vi "F Dwf Analog Out Amplitude Info.vi"(7 "pvoltsMax":dbl, 8 "error in (no error)":errorcluster, 9 "pvoltsMin":dbl, 10 "idxChannel":i32, 11 "hdwf":i32) -> (0 "error out":errorcluster, 1 "pvoltsMin out":dbl, 3 "function return":i32, 5 "pvoltsMax out":dbl)   [LabVIEW 2019, in "Olasdwf.lvlib"]
doc: "DWFAPI int FDwfAnalogOutAmplitudeInfo(HDWF hdwf, int idxChannel, double *pvoltsMin, double *pvoltsMax);"
uses:
  Olasdwf.lvlib
  Windows/System32/dwf.dll
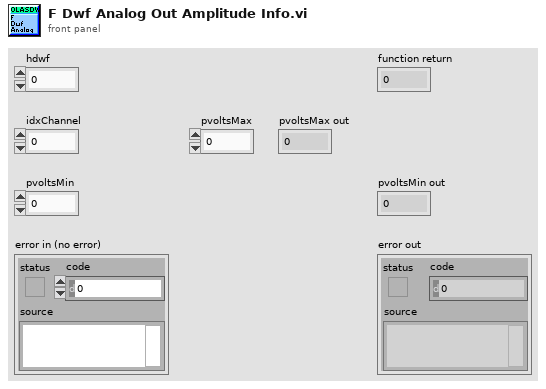
[diagram p1: front panel]
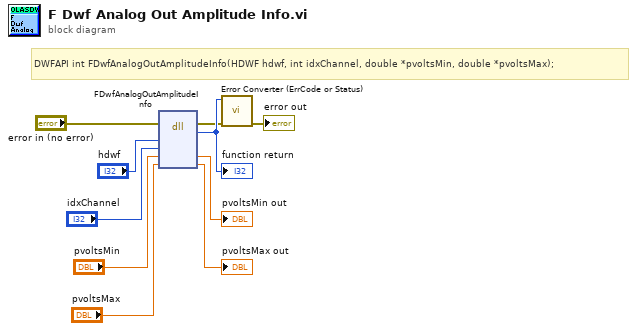
[diagram p0: block diagram]
diagram:
  # "DWFAPI int FDwfAnalogOutAmplitudeInfo(HDWF hdwf, int idxChannel, double *pvoltsMin, double *pvoltsMax);"
  n1 = dll-call lib="C:/Windows/System32/dwf.*" fn="FDwfAnalogOutAmplitudeInfo"(error in="error in (no error)", "hdwf"="hdwf", "idxChannel"="idxChannel", "pvoltsMin"="pvoltsMin", "pvoltsMax"="pvoltsMax") -> (error out=w2:errorcluster, w10:i32, "pvoltsMin"=→"pvoltsMin out":dbl, "pvoltsMax"=→"pvoltsMax out":dbl)  [unwired: 4 in, 1 out]
  "function return" <- w10
  n2 = call "Error Converter (ErrCode or Status).vi"("error in (no error)"=w2, "error code"=w10) -> ("error out"=→"error out":errorcluster)  [unwired: 9 in]
